vi "[Generate Test Cases] File or directory exists.vi"(11 "Targets":T1(array[cluster])) -> (3 "Test Cases":refnum<class "TestCase.lvclass">[](array[class]))   [LabVIEW 2016, in "Tests.lvlib" / "[Test Suite] File Transfer Behavior.lvclass"]
uses:
  [Test Suite] File Transfer Behavior.lvclass
  <vilib>/addons/_JKI Toolkits/VI Tester/TestCase.llb/TestCase.lvclass
  classes/FTP/FTP.lvclass
  C:/GitHub/SystemManagementAndInformation/source/classes/File Transfer Behavior/File Transfer Behavior.lvclass
  classes/WebDAV/WebDAV.lvclass
  classes/File Transfer Behavior/File Transfer Behavior.lvclass
  classes/File Transfer Behavior/File Transfer Behavior.lvclass/File Transfer Behavior.ctl
  [Test Case] File or directory exists/[Test Case] File or directory exists.lvclass
  C:/Program Files (x86)/National Instruments/LabVIEW 2016/vi.lib/addons/_JKI Toolkits/VI Tester/TestCase.llb/TestCase.lvclass
  [Test Case] File or directory exists/[Test Case] File or directory exists.lvclass/[Test Case] File or directory exists.ctl
  [Test Case] File or directory exists/Write File Transfer Behavior.lvclass.vi
  [Test Case] File or directory exists/Write Path to test.vi
  [Test Case] File or directory exists/Write Expected result.vi
  classes/File Transfer Behavior/Set Address.vi
  classes/File Transfer Behavior/Set Password.vi
  classes/File Transfer Behavior/Set Username.vi
  classes/RT Management/RT Management.lvclass
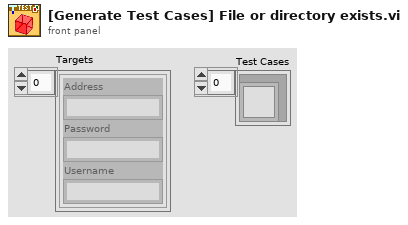
[diagram p1: front panel]
types:
  T1 = cluster{"Address":string, "Password":string, "Username":string}[]
  T2 = cluster{"Path to test":string, "Expected result":bool}[]
  T3 = cluster{"Path to test":string, "Expected result":bool}
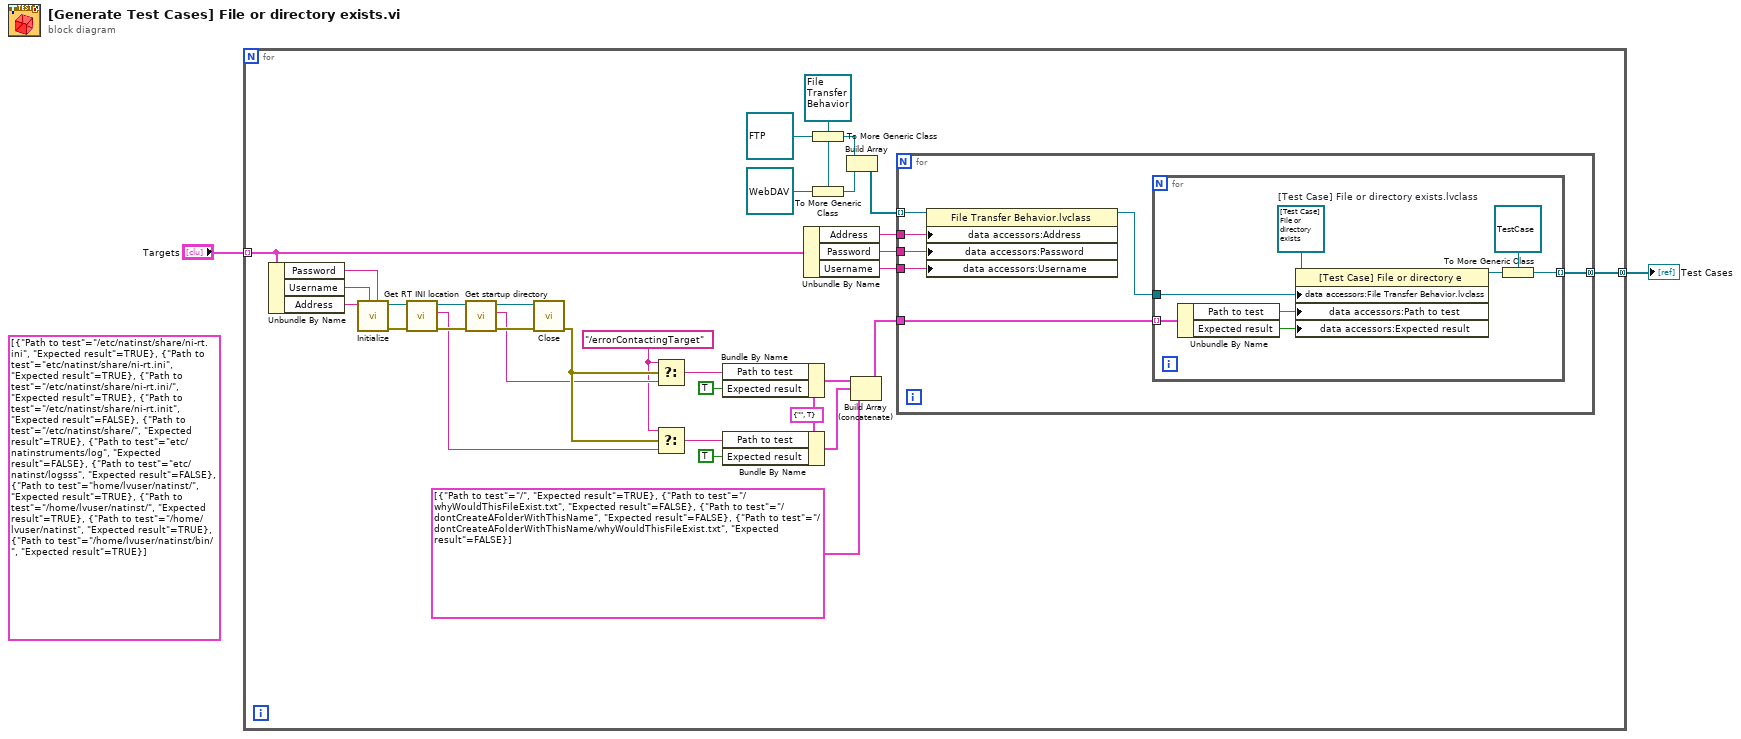
[diagram p0: block diagram]
diagram:
  (unwired) T2 [{"Path to test"="/etc/natinst/share/ni-rt.ini", "Expected result"=TRUE}, {"Path to test"="etc/natinst/share/ni-rt.ini", "Expected result"=TRUE}, {"Path to test"="/etc/natinst/share/ni-rt.ini/", "Expected result"=TRUE}, {"Path to test"="/etc/natinst/share/ni-rt.init", "Expected result"=FALSE}, {"Path to test"="/etc/natinst/share/", "Expected result"=TRUE}, {"Path to test"="etc/natinstruments/log", "Expected result"=FALSE}, {"Path to test"="etc/natinst/logsss", "Expected result"=FALSE}, {"Path to test"="home/lvuser/natinst/", "Expected result"=TRUE}, {"Path to test"="/home/lvuser/natinst/", "Expected result"=TRUE}, {"Path to test"="/home/lvuser/natinst", "Expected result"=TRUE}, {"Path to test"="/home/lvuser/natinst/bin/", "Expected result"=TRUE}]
  n1 = for {
    tunnel: [w35] -> w2 mode=concatenating
    tunnel: "Targets" -> [w25] mode=indexing
    w3 = "/errorContactingTarget" ("t")
    w17 = T3 {"Path to test"="", "Expected result"=TRUE}
    w34 = refnum<class "File Transfer Behavior.lvclass"> refnum ("RT Management.lvlib:File Transfer Behavior.lvclass")
    n2 = Unbundle By Name(w25) -> ("Password"=w22:string, "Username"=w23:string, "Address"=w24:string)
    n3 = call "Initialize.vi"("Password"=w22, "Username (\"\" : target default)"=w23, "Target"=w24) -> ("error out"=w15:errorcluster, "RT Management out"=w16:refnum<class "RT Management.lvclass">)  [unwired: 6 in, 1 out]
    n4 = call "Get RT INI location.vi"("error in (no error)"=w15, "RT Management in"=w16) -> ("error out"=w14:errorcluster, "RT INI Location"=w4:string, "RT Management out"=w13:refnum<class "RT Management.lvclass">)  [unwired: 7 in]
    n5 = call "Get startup directory.vi"("error in (no error)"=w14, "RT Management in"=w13) -> ("error out"=w12:errorcluster, "Startup directory"=w5:string, "RT Management out"=w11:refnum<class "RT Management.lvclass">)  [unwired: 7 in]
    n6 = call "Close.vi"("error in (no error)"=w12, "RT Management in"=w11) -> ("error out"=w6:errorcluster)  [unwired: 9 in]
    n7 = Select(t=w3, s=w6, f=w5) -> (s? t:f=w8:string)
    n8 = Select(t=w3, s=w6, f=w4) -> (s? t:f=w7:string)
    n9 = Bundle By Name(cluster=w17, "Path to test"=w8, "Expected result"=TRUE) -> (w19:T3)
    n10 = Bundle By Name(cluster=w17, "Path to test"=w7, "Expected result"=TRUE) -> (w18:T3)
    n11 = Unbundle By Name(w25) -> ("Address"=w28:string, "Password"=w27:string, "Username"=w26:string)
    n12 = To More Generic Class(target class=w34, reference=refnum<class "FTP.lvclass"> refnum ("RT Management.lvlib:FTP.lvclass")) -> (generic class reference=w31:refnum<class "File Transfer Behavior.lvclass">)
    n13 = To More Generic Class(target class=w34, reference=refnum<class "WebDAV.lvclass"> refnum ("RT Management.lvlib:WebDAV.lvclass")) -> (generic class reference=w30:refnum<class "File Transfer Behavior.lvclass">)
    n14 = Build Array(w31, w30) -> (w29:refnum<class "File Transfer Behavior.lvclass">[])
    n15 = Build Array (concatenate)(w19, w18, T2 [{"Path to test"="/", "Expected result"=TRUE}, {"Path to test"="/whyWouldThisFileExist.txt", "Expected result"=FALSE}, {"Path to test"="/dontCreateAFolderWithThisName", "Expected result"=FALSE}, {"Path to test"="/dontCreateAFolderWithThisName/whyWouldThisFileExist.txt", "Expected result"=FALSE}]) -> (w20:T2)
    n16 = for {
      tunnel: w28 -> [w41]
      tunnel: w27 -> [w40]
      tunnel: w26 -> [w39]
      tunnel: w20 -> [w38]
      tunnel: [w37] -> w35 mode=concatenating
      tunnel: w29 -> [w36] mode=indexing
      n17 = property class="File Transfer Behavior.lvclass"(reference=w36, "data accessors:Address"=w41, "data accessors:Password"=w40, "data accessors:Username"=w39) -> (reference out=w42:refnum<class "File Transfer Behavior.lvclass">)  [unwired: 1 in, 1 out]
      n18 = for {
        tunnel: w42 -> [w49]
        tunnel: w38 -> [w48] mode=indexing
        tunnel: [w43] -> w37 mode=indexing
        w50 = refnum<class "[Test Case] File or directory exists.lvclass"> refnum  # [Test Case] File or directory exists.lvclass
        n19 = Unbundle By Name(w48) -> ("Path to test"=w47:string, "Expected result"=w46:bool)
        n20 = property class="[Test Case] File or directory e"(reference=w50, "data accessors:File Transfer Behavior.lvclass"=w49, "data accessors:Path to test"=w47, "data accessors:Expected result"=w46) -> (reference out=w45:refnum<class "[Test Case] File or directory exists.lvclass">)  [unwired: 1 in, 1 out]
        n21 = To More Generic Class(target class=refnum<class "TestCase.lvclass"> refnum ("TestCase.lvclass"), reference=w45) -> (generic class reference=w43:refnum<class "TestCase.lvclass">)
      }
    }
  }
  "Test Cases" <- w2
